vi "Project_1.vi"() -> ()   [LabVIEW 2018]
uses:
  <vilib>/Instr/_visa.llb/VISA Configure Serial Port (Instr).vi
panel:
  out "?":bool
  in  "发送":string
  in  "接收区":string
  in  "停止":bool
  in  "清空":bool
  in  "发送":bool
  in  "打开":bool
  out "奇偶校验\n停止位 3":dbl
  out "数据位\n停止位 2":dbl
  out "停止位\n停止位":dbl
  out "波特率":dbl
  out "串口选择":string
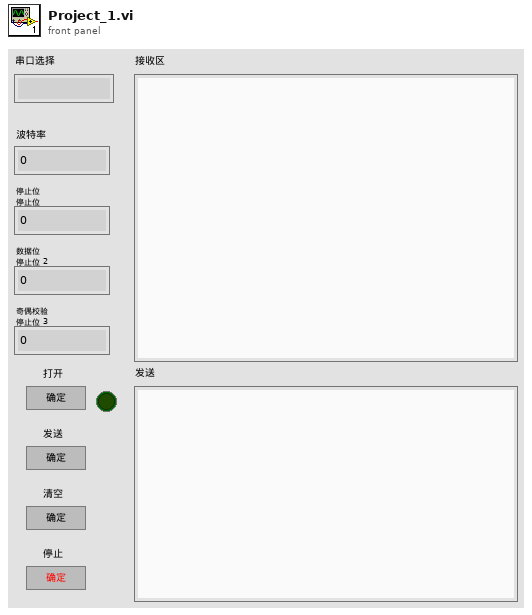
[diagram p1: front panel]
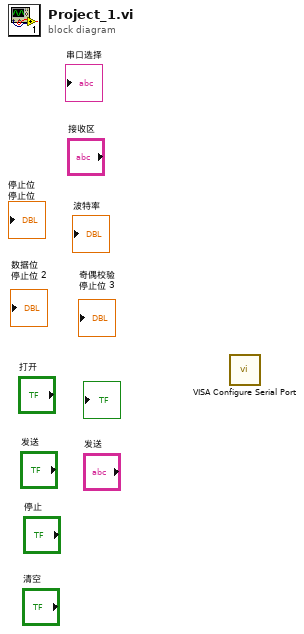
[diagram p0: block diagram]
diagram:
  n1 = call-poly "VISA Configure Serial Port"() -> ()  [unwired: 14 in, 2 out]
